vi "Corner Detect.vi"() -> ()   [LabVIEW 2016]
uses:
  <vilib>/vision/NI_Vision_Development_Module.lvlib
panel:
  out "IMG2":T1(plugin-control)
  in  "Feature descriptor":enum32{"FREAK", "BRISK"}(ring)
  in  "Method":enum16{"Harris", "Shi-Tomasi", "FAST"}(ring)=enum."FAST"
  out "TMP":T1(plugin-control)
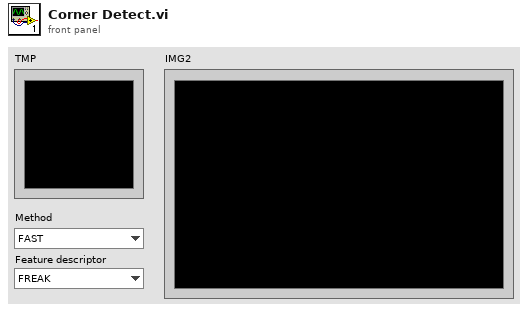
[diagram p1: front panel]
types:
  T1 = typedef "IMAQ Image.ctl" = refnum<image>
  T2 = cluster{"Detector type":enum32{"Harris Corner", "Shi-Tomasi Corner"}, "Kernel size":i32, "Min Corner Point Strength":dbl}
  T3 = cluster{"Image 1":cluster{"X":sgl, "Y":sgl}, "Image2":cluster{"X":sgl, "Y":sgl}}[]
  T4 = cluster{"X Resolution":i32, "Y Resolution":i32}[]
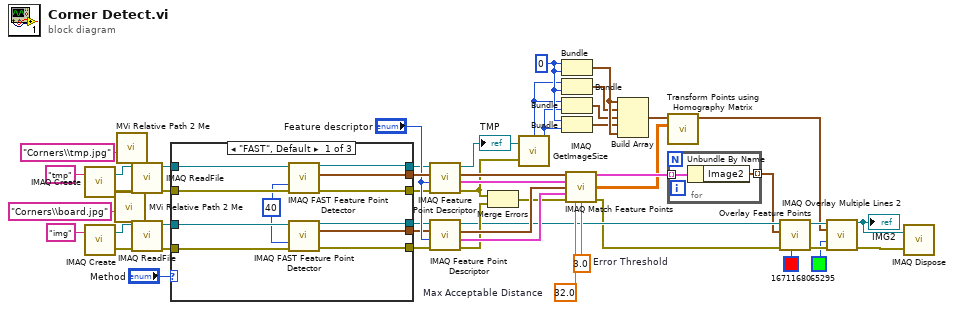
[diagram p0: block diagram]
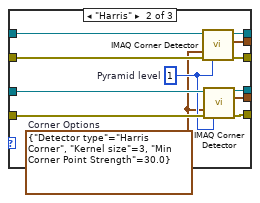
[diagram p2: hidden frame]
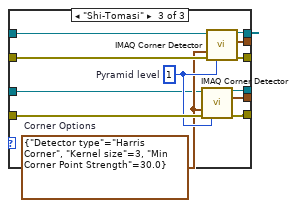
[diagram p3: hidden frame]
diagram:
  w30 = 3.0  # Error Threshold
  w31 = 32.0  # Max Acceptable Distance
  w17 = 0
  n1 = call "IMAQ Create"("Image Name"="tmp") -> ("Src"=w51:T1, "error out"=w52:errorcluster)  [unwired: 4 in]
  n2 = call "IMAQ Create"("Image Name"="img") -> ("Src"=w41:T1, "error out"=w43:errorcluster)  [unwired: 4 in]
  n3 = call "MVi Relative Path 2 Me.vi"("Relative Path"="Corners\\board.jpg" ("name or relative path")) -> ("Appended Dir"=w39:path)  [unwired: 5 in, 1 out]
  n4 = call "MVi Relative Path 2 Me.vi"("Relative Path"="Corners\\tmp.jpg" ("name or relative path")) -> ("Appended Dir"=w48:path)  [unwired: 5 in, 1 out]
  n5 = call "IMAQ ReadFile"("File Path"=w48, "error in (no error)"=w52, "Image"=w51) -> ("error out"=w46:errorcluster, "Image Out"=w45:T1)  [unwired: 4 in, 3 out]
  n6 = call "IMAQ ReadFile"("File Path"=w39, "error in (no error)"=w43, "Image"=w41) -> ("error out"=w2:errorcluster, "Image Out"=w3:T1)  [unwired: 4 in, 3 out]
  n7 = case shown="\"FAST\", Default" "Method" {
    tunnel: w45 -> [w62 w74 w86]
    tunnel: w46 -> [w63 w75 w87]
    tunnel: [w61 w73 w85] -> w7
    tunnel: [w60 w72 w84] -> w6
    tunnel: [w59 w71 w83] -> w44
    tunnel: w2 -> [w58 w68 w82]
    tunnel: w3 -> [w57 w67 w76]
    tunnel: [w56 w69 w81] -> w28
    tunnel: [w55 w70 w79] -> w29
    tunnel: [w54 w64 w80] -> w37
    frame "FAST", Default {
      w53 = 40 ("Min Feature Point Strength")
      n8 = call "IMAQ FAST Feature Point Detector"("Image"=w62, "Min Feature Point Strength"=w53, "error in (no error)"=w63) -> ("Image (duplicate)"=w61:T1, "Feature Point Coordinates"=w59:cluster{"X":sgl, "Y":sgl}[], "error out"=w60:errorcluster)  [unwired: 7 in, 3 out]
      n9 = call "IMAQ FAST Feature Point Detector"("Image"=w57, "Min Feature Point Strength"=w53, "error in (no error)"=w58) -> ("Image (duplicate)"=w55:T1, "Feature Point Coordinates"=w54:cluster{"X":sgl, "Y":sgl}[], "error out"=w56:errorcluster)  [unwired: 7 in, 3 out]
    }
    frame "Harris" {
      w66 = u32 1  # Pyramid level
      w65 = T2 {"Detector type"=enum."Harris Corner", "Kernel size"=3, "Min Corner Point Strength"=30.0}  # Corner Options
      n10 = call "IMAQ Corner Detector"("Image"=w74, "Corner Options"=w65, "error in (no error)"=w75, "Pyramid level"=w66) -> ("Image (duplicate)"=w73:T1, "Corner Point Coordinates"=w71:cluster{"X":sgl, "Y":sgl}[], "error out"=w72:errorcluster)  [unwired: 6 in, 3 out]
      n11 = call "IMAQ Corner Detector"("Image"=w67, "Corner Options"=w65, "error in (no error)"=w68, "Pyramid level"=w66) -> ("Image (duplicate)"=w70:T1, "Corner Point Coordinates"=w64:cluster{"X":sgl, "Y":sgl}[], "error out"=w69:errorcluster)  [unwired: 6 in, 3 out]
    }
    frame "Shi-Tomasi" {
      w77 = T2 {"Detector type"=enum."Harris Corner", "Kernel size"=3, "Min Corner Point Strength"=30.0}  # Corner Options
      w78 = u32 1  # Pyramid level
      n12 = call "IMAQ Corner Detector"("Image"=w76, "Corner Options"=w77, "error in (no error)"=w82, "Pyramid level"=w78) -> ("Image (duplicate)"=w79:T1, "Corner Point Coordinates"=w80:cluster{"X":sgl, "Y":sgl}[], "error out"=w81:errorcluster)  [unwired: 6 in, 3 out]
      n13 = call "IMAQ Corner Detector"("Image"=w86, "Corner Options"=w77, "error in (no error)"=w87, "Pyramid level"=w78) -> ("Image (duplicate)"=w85:T1, "Corner Point Coordinates"=w83:cluster{"X":sgl, "Y":sgl}[], "error out"=w84:errorcluster)  [unwired: 6 in, 3 out]
    }
  }
  n14 = call "IMAQ Feature Point Descriptor"("error in (no error)"=w6, "Feature descriptor method"="Feature descriptor", "Feature Point Coordinates In"=w44, "Image"=w7) -> ("error out"=w1:errorcluster, "Feature Descriptors"=w34:cluster{"Descriptor":u8[]}[], "Feature Point Coordinates Out"=w36:cluster{"X":sgl, "Y":sgl}[], "Image (duplicate)"=w13:T1)  [unwired: 4 in]
  "TMP" <- w13
  n15 = call "IMAQ Feature Point Descriptor"("error in (no error)"=w28, "Feature descriptor method"="Feature descriptor", "Feature Point Coordinates In"=w37, "Image"=w29) -> ("error out"=w32:errorcluster, "Feature Descriptors"=w33:cluster{"Descriptor":u8[]}[], "Feature Point Coordinates Out"=w35:cluster{"X":sgl, "Y":sgl}[], "Image (duplicate)"=w26:T1)  [unwired: 4 in]
  n16 = Merge Errors(w1, w32) -> (w12:errorcluster)
  n17 = call "IMAQ GetImageSize"("Image"=w13, "error in (no error)"=w1) -> ("Y Resolution"=w10:i32, "X Resolution"=w11:i32)  [unwired: 2 in, 1 out]
  n18 = Bundle(w17, w17) -> (w18:cluster{i32, i32})  [unwired: 1 in]
  n19 = Bundle("X Resolution"=w11, w17) -> (w14:cluster{"X Resolution":i32, i32})  [unwired: 1 in]
  n20 = Bundle("X Resolution"=w11, "Y Resolution"=w10) -> (w15:cluster{"X Resolution":i32, "Y Resolution":i32})  [unwired: 1 in]
  n21 = Bundle(w17, "Y Resolution"=w10) -> (w16:cluster{i32, "Y Resolution":i32})  [unwired: 1 in]
  n22 = call "IMAQ Match Feature Points"("Feature Points 1"=w36, "Feature Descriptors 1"=w34, "Feature Points  2"=w35, "Feature Descriptors 2"=w33, "error in (no error)"=w12, "Max Acceptable Distance"=w31, "Error Threshold"=w30) -> ("Match Locations"=w27:T3, "Homography Matrix"=w23:dbl[][], "error out"=w25:errorcluster)  [unwired: 5 in, 1 out]
  n23 = Build Array(w18, w14, w15, w16, w18) -> (w9:T4)
  n24 = call "Transform Points using Homography Matrix.vi"("Homography Matrix"=w23, "Points"=w9) -> ("Transformed Points"=w4:cluster{"X":dbl, "Y":dbl}[])  [unwired: 9 in]
  n25 = for {
    tunnel: w27 -> [w89] mode=indexing
    tunnel: [w88] -> w24 mode=indexing
    n26 = Unbundle By Name(w89) -> ("Image2"=w88:cluster{"X":sgl, "Y":sgl})
  }
  n27 = call "Overlay Feature Points.vi"("Color"=u32 16711680, "error in"=w25, "Feature Points"=w24, "Image"=w26) -> ("error out"=w21:errorcluster, "Image Out"=w22:T1)  [unwired: 6 in]
  n28 = call "IMAQ Overlay Multiple Lines 2"("Image"=w22, "Line End Points"=w4, "Color"=u32 65295, "error in (no error)"=w21) -> ("Image Out"=w19:T1, "error out"=w20:errorcluster)  [unwired: 10 in]
  "IMG2" <- w19
  n29 = call "IMAQ Dispose"("Image"=w19, "error in (no error)"=w20) -> ()  [unwired: 4 in, 1 out]
